vi "LibXML_NavigateNode.vi"(4 "error in (no error)":errorcluster, 5 "direction":T1, 6 "node in":u32) -> (0 "error out":errorcluster, 2 "blankNode":bool, 3 "node out":u32)   [LabVIEW 2019, in "Tools.lvlib" / "LibXML.lvlib"]
doc: "Get another node relative to the input node."
uses:
  LibXML.lvlib
  LibXML_NavigateDirection.ctl
  dll/lXMLwrap.dll
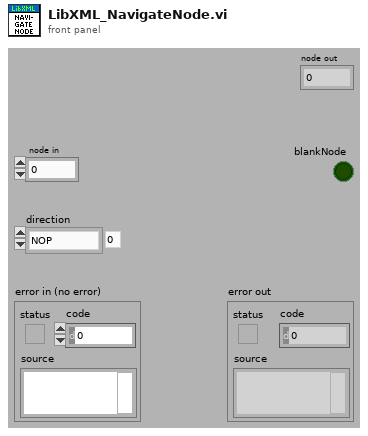
[diagram p1: front panel]
types:
  T1 = typedef "Tools.lvlib/LibXML.lvlib/LibXML_NavigateDirection.ctl" = enum16{"NOP", "first child", "last child", "parent", "next", "prev"}
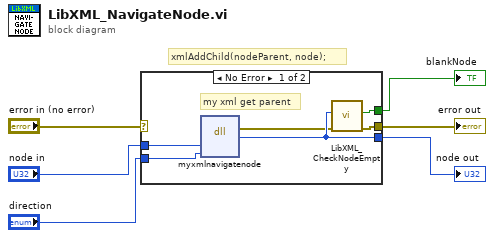
[diagram p0: block diagram]
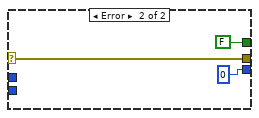
[diagram p2: hidden frame]
diagram:
  # "xmlAddChild(nodeParent, node);"
  n1 = case shown="No Error" "error in (no error)" {
    selector: "error in (no error)" -> [_ w15]
    tunnel: [w10 w15] -> w5
    tunnel: "node in" -> [w12 _]
    tunnel: "direction" -> [w11 _]
    tunnel: [w9 FALSE ("blankNode!")] -> w2
    tunnel: [w8 u32 0 ("return type")] -> w1
    frame No Error {
      # "my xml get parent"
      n2 = dll-call lib="C:/Projects/_Prywatne/MyCIT/Framework/Tools/XML/LibXML/dll/lXMLwrap.dll" fn="myxmlnavigatenode"("node"=w12, "type"=w11) -> (error out=w7:errorcluster, "return type"=w8:u32)  [unwired: 5 in, 1 out]
      n3 = call "LibXML_CheckNodeEmpty.vi"("error in"=w7, "node in"=w8) -> ("error out"=w10:errorcluster, "blankNode!"=w9:bool)  [unwired: 8 in]
    }
    frame Error {
    }
  }
  "error out" <- w5
  "blankNode" <- w2
  "node out" <- w1
